vi "Add infinitesimal to Double.vi"(1 "DBL (x)":dbl) -> (0 "Dual (x+e)":refnum<class "Dual.lvclass">)   [LabVIEW 2020, in "Automatic Differentiation.lvlib" / "Dual.lvclass"]
uses:
  Dual.lvclass
  Dual.lvclass/Dual.ctl
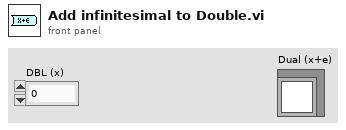
[diagram p1: front panel]
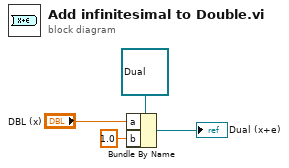
[diagram p0: block diagram]
diagram:
  n1 = Bundle By Name(cluster=refnum<class "Dual.lvclass"> refnum ("Dual out"), "a"="DBL (x)", "b"=1.0) -> (→"Dual (x+e)":refnum<class "Dual.lvclass">)
